vi "Draw GPR Graph.vi"(6 "Draw Area Size":cluster{"Width":u32, "Height":u32}, 7 "Graph Info":T1 caption="State", 8 "error in":errorcluster, 11 "Data":dbl[][](array[numeric])) -> (0 "error out":errorcluster, 3 "picture out":picture)   [LabVIEW 2009]
doc: "Given Display Information, a 2-D array of data, and the size of a picture control, this VI draws a GPR graph and returns it as a picture control."
uses:
  Controls/GPR Graph Info.ctl
  Controls/Display Types.ctl
  Controls/Display Info.ctl
  Controls/Trace Options.ctl
  Controls/Fill Options.ctl
  Controls/Intensity Options.ctl
  Controls/Color Scales.ctl
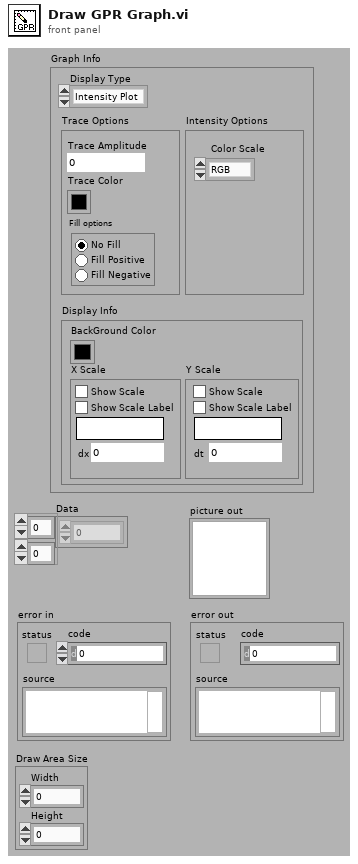
[diagram p1: front panel]
types:
  T1 = typedef "GPR Graph Info.ctl" = cluster{"Display Type":T2, "Display Info":T3, "Trace Options":T4, "Intensity Options":T6}
  T2 = typedef "Display Types.ctl" = enum16{"Intensity Plot", "Wiggle Trace"}
  T3 = typedef "Display Info.ctl" = cluster{"X Scale":cluster{"X Scale Label":bool, "X Scale Name":string, "X Scale Visible":bool, "dx":dbl}, "Y Scale":cluster{"X Scale Label":bool, "X Scale Name":string, "X Scale Visible":bool, "dt":dbl}, "BackGround Color":u32}
  T4 = typedef "Trace Options.ctl" = cluster{"Trace Amplitude":dbl, "Trace Color":u32, "Fill options":T5}
  T5 = typedef "Fill Options.ctl" = enum32{"No Fill", "Fill Positive", "Fill Negative"}
  T6 = typedef "Intensity Options.ctl" = cluster{"Color Scale":T7}
  T7 = typedef "Color Scales.ctl" = enum16{"RGB", "RWB", "BGR", "BWR", "BW", "WB"}
  T8 = cluster{"left":i16, "top":i16, "right":i16, "bottom":i16}
  T9 = typedef "imagedata.ctl" = cluster{"image type":i32, "image depth":i32, "image":u8[], "mask":u8[], "colors":u32[], "Rectangle":cluster{"left":i16, "top":i16, "right":i16, "bottom":i16}}
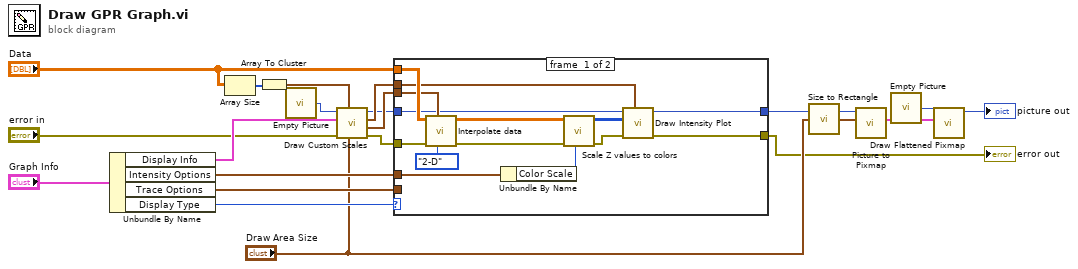
[diagram p0: block diagram]
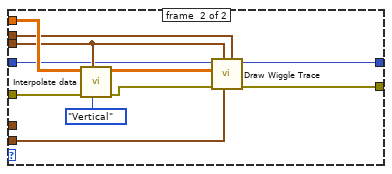
[diagram p2: hidden frame]
diagram:
  n1 = Unbundle By Name("Graph Info") -> ("Display Info"=w19:T3, "Intensity Options"=w20:T6, "Trace Options"=w17:T4, "Display Type"=w18:T2)
  n2 = Array Size(array="Data") -> (size(s)=w9:i32[])
  n3 = Array To Cluster(array=w9) -> (cluster=w15:cluster{"[0]":i32, "[1]":i32})
  n4 = call "Empty Picture"() -> ("empty picture"=w21:picture)
  n5 = call "Draw Custom Scales.vi"("Draw Area Size"="Draw Area Size", "Number of Points"=w15, "error in"="error in", "Custom Graph Info"=w19, "picture in"=w21) -> ("error out"=w8:errorcluster, "Plot Area Size"=w14:cluster{"Width":u32, "Height":u32}, "Offsets"=w13:cluster{"X offset":u32, "Y offset":u32}, "picture out"=w12:picture)  [unwired: 3 in]
  n6 = case shown="\"Wiggle Trace\"" w18 {
    tunnel: w13 -> [w29 w41]
    tunnel: "Data" -> [w35 w44]
    tunnel: w8 -> [w33 w43]
    tunnel: [w32 w42] -> w5
    tunnel: w14 -> [w30 w40]
    tunnel: [w28 w36] -> w1
    tunnel: w12 -> [w26 w39]
    tunnel: w17 -> [_ w38]
    tunnel: w20 -> [w25 _]
    frame #0 {
      n7 = call "Interpolate data.vi"("Interpolation Direction"=enum16{"Horizontal", "Vertical", "2-D"}."2-D", "Draw Area Size"=w30, "error in"=w33, "Data"=w35) -> ("error out"=w31:errorcluster, "Resampled Data"=w34:dbl[][])  [unwired: 6 in]
      n8 = Unbundle By Name(w25) -> ("Color Scale"=w24:T7)
      n9 = call "Scale Z values to colors.vi"("Scale"=w24, "error in"=w31, "Values"=w34) -> ("error out"=w22:errorcluster, "Colors"=w27:u32[][])  [unwired: 6 in, 1 out]
      n10 = call "Draw Intensity Plot.vi"("Offsets"=w29, "error in"=w22, "Data"=w27, "picture in"=w26) -> ("error out"=w28:errorcluster, "picture out"=w32:picture)  [unwired: 6 in]
    }
    frame #1 {
      n11 = call "Interpolate data.vi"("Interpolation Direction"=enum16{"Horizontal", "Vertical", "2-D"}."Vertical", "Draw Area Size"=w40, "error in"=w43, "Data"=w44) -> ("error out"=w46:errorcluster, "Resampled Data"=w45:dbl[][])  [unwired: 6 in]
      n12 = call "Draw Wiggle Trace.vi"("Offsets"=w41, "Trace Options"=w38, "Plot Area Size"=w40, "error in (no error)"=w46, "Data"=w45, "picture in"=w39) -> ("error out"=w36:errorcluster, "picture out"=w42:picture)  [unwired: 4 in]
    }
  }
  "error out" <- w1
  n13 = call "Size to Rectangle.vi"("Size"="Draw Area Size") -> ("rect"=w6:T8)
  n14 = call <vilib>:"Picture to Pixmap.vi"("rect"=w6, "picture"=w5) -> ("image data"=w4:T9)  [unwired: 8 in, 1 out]
  n15 = call "Empty Picture"() -> ("empty picture"=w3:picture)
  n16 = call <vilib>:"Draw Flattened Pixmap.vi"("image data"=w4, "picture"=w3) -> ("new picture"=→"picture out":picture)  [unwired: 7 in]
